vi "OSU100_Connect.vi"(8 "error in (no error)":errorcluster, 9 "DeviceName":string) -> (0 "error out":errorcluster, 3 "Reference out":refnum<k24>)   [LabVIEW 2017]
uses:
  C:/Users/Ssantec_Test/Documents/Instrument_DLL_Sample_Labview_20220902_Ver1.2.2/DLL/x86/InstrumentDLL.dll
  DLL/x86/InstrumentDLL.dll
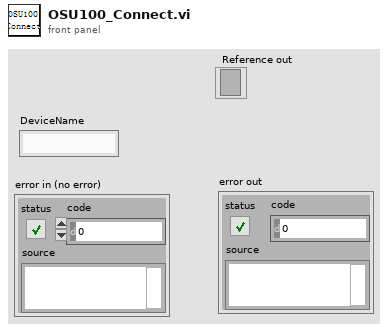
[diagram p1: front panel]
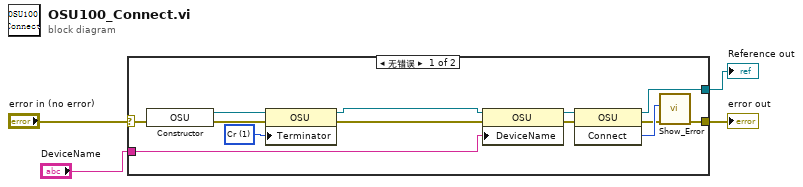
[diagram p0: block diagram]
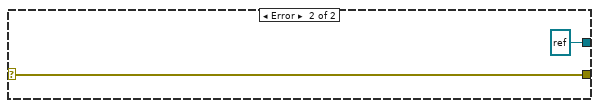
[diagram p2: hidden frame]
diagram:
  n1 = case shown="无错误" "error in (no error)" {
    selector: "error in (no error)" -> [w8 w19]
    tunnel: "DeviceName" -> [w7 _]
    tunnel: [w17 refnum<k24> refnum ("new reference")] -> w3
    tunnel: [w14 w19] -> w1
    frame No Error {
      w11 = 1 items=["CrLf", "Cr", "Lf"] ("Terminator")
      n2 = constructor class="OSU"(error in=w8) -> (reference out=w13:refnum<k24>, error out=w12:errorcluster)  [unwired: 2 in, 1 out]
      n3 = property on="属性节点" class="OSU"(reference=w13, error in=w12, "Terminator"=w11) -> (reference out=w10:refnum<k24>, error out=w6:errorcluster)
      n4 = property on="属性节点" class="OSU"(reference=w10, error in=w6, "DeviceName"=w7) -> (reference out=w9:refnum<k24>, error out=w5:errorcluster)
      n5 = invoke on="调用节点" class="OSU" method="Connect"(reference=w9, error in=w5) -> (reference out=w17:refnum<k24>, error out=w15:errorcluster, "Connect"=w16:i32)  [unwired: 1 in]
      n6 = call "Show_Error.vi"("error in (no error)"=w15, "Error"=w16) -> ("error out"=w14:errorcluster)  [unwired: 9 in]
    }
    frame Error {
    }
  }
  "error out" <- w1
  "Reference out" <- w3
